vi "loadDataIntoScript.vi"(8 "error in (no error)":errorcluster, 9 "Path":path=path "C:/Users/Administrator/Desktop/Crete/Lua/Sweeping/lvScript.tsp", 10 "data":dbl[][][](array[numeric]), 11 "K2602 in":refnum<class "K2602.lvclass">) -> (0 "error out":errorcluster, 2 "script":string, 3 "K2602 out":refnum<class "K2602.lvclass">)   [LabVIEW 2011, in "Hardware.lvlib" / "Channels.lvlib" / "K2602.lvclass"]
uses:
  K2602.lvclass
  K2602.lvclass/K2602.ctl
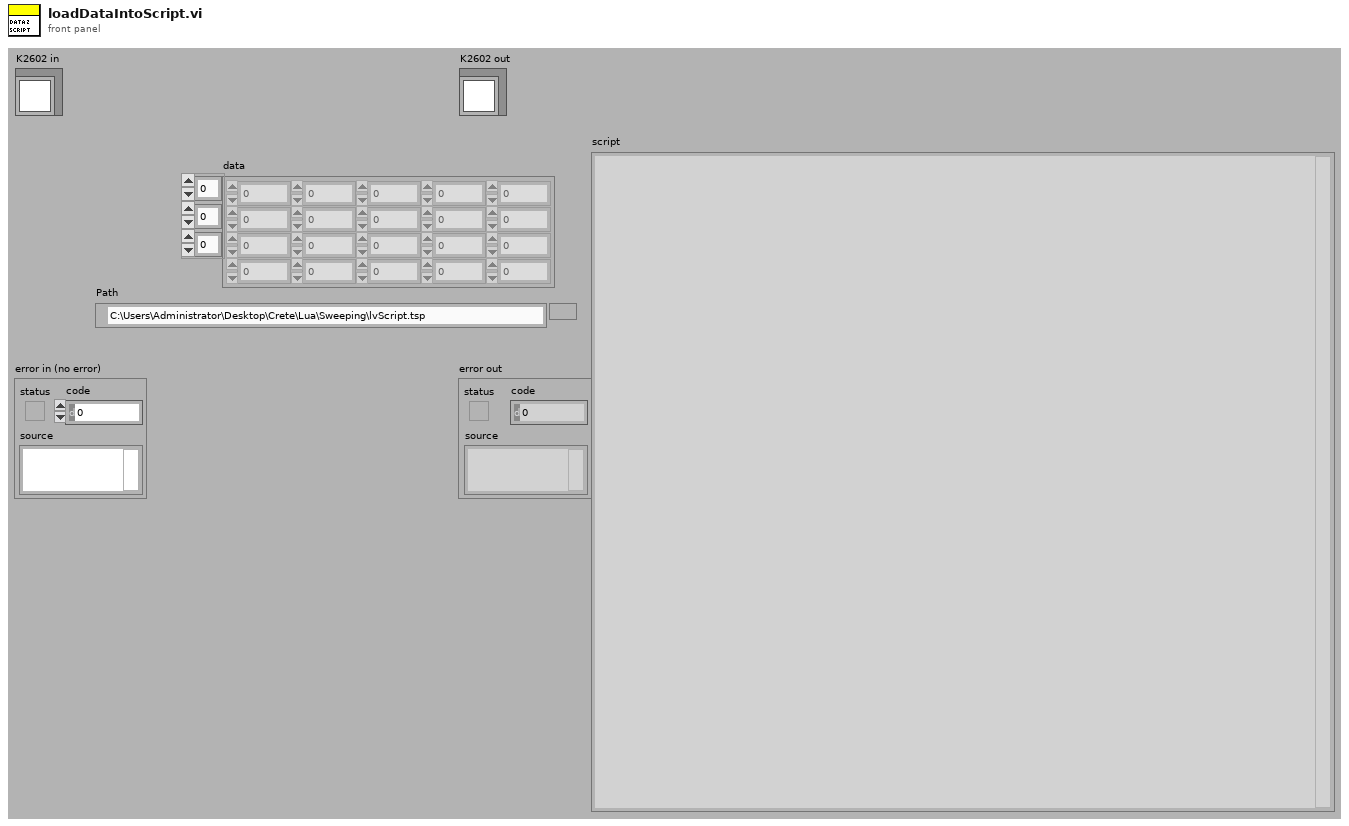
[diagram p1: front panel]
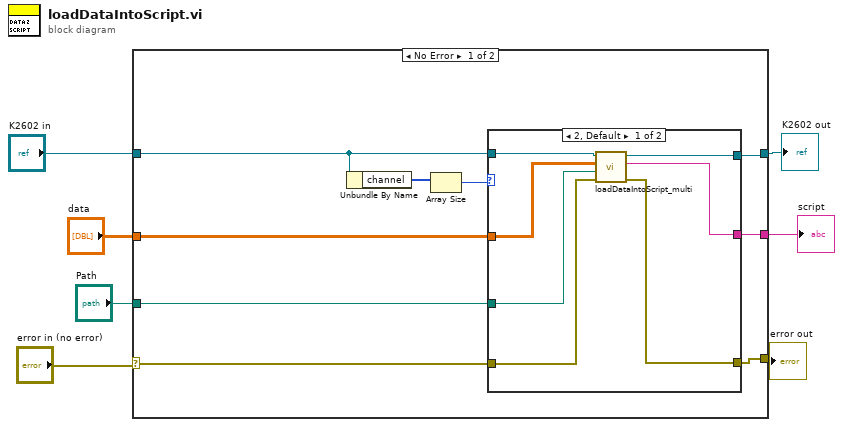
[diagram p0: block diagram]
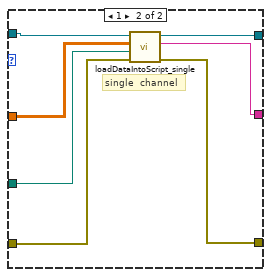
[diagram p2: hidden frame]
diagram:
  n1 = case shown="No Error" "error in (no error)" {
    selector: "error in (no error)" -> [w15 w32]
    tunnel: [w14 w32] -> w6
    tunnel: [w16 w31] -> w2
    tunnel: "K2602 in" -> [w10 w31]
    tunnel: "data" -> [w12 _]
    tunnel: "Path" -> [w11 _]
    tunnel: [w13 _] -> w1
    frame No Error {
      n2 = Unbundle By Name(w10) -> ("channel"=w9:i32[])
      n3 = Array Size(array=w9) -> (size(s)=w8:i32)
      n4 = case shown="2, Default" w8 {
        tunnel: w10 -> [w23 w30]
        tunnel: [w22 w29] -> w16
        tunnel: w15 -> [w20 w28]
        tunnel: [w19 w27] -> w14
        tunnel: [w18 w26] -> w13
        tunnel: w12 -> [w21 w25]
        tunnel: w11 -> [w17 w24]
        frame 2, Default {
          n5 = call "loadDataIntoScript_multi.vi"("error in (no error)"=w20, "Path"=w17, "data"=w21, "K2602 in"=w23) -> ("error out"=w19:errorcluster, "script"=w18:string, "K2602 out"=w22:refnum<class "K2602.lvclass">)  [unwired: 5 in]
        }
        frame 1 {
          # "single  channel"
          n6 = call "loadDataIntoScript_single.vi"("error in (no error)"=w28, "Path"=w24, "data"=w25, "K2602 in"=w30) -> ("error out"=w27:errorcluster, "script"=w26:string, "K2602 out"=w29:refnum<class "K2602.lvclass">)  [unwired: 5 in]
        }
      }
    }
    frame Error {
    }
  }
  "error out" <- w6
  "K2602 out" <- w2
  "script" <- w1
